vi "DetermineSpeedCap.vi"(2 "Speed Cap Decceleration Limit (/s)":dbl=0.25, 3 "Driver Profile Doesn't Want to Shift":bool, 4 "Master State":T1(ring)) -> (0 "Speed Cap [0,1]":dbl)   [LabVIEW 2020]
doc: "Determines the speed cap for the swerve drive based on the control inputs and master alarms. This includes forcing the robot into low gear."
uses:
  GlobalDriverStationCommands.vi
  GlobalDrivebase.vi
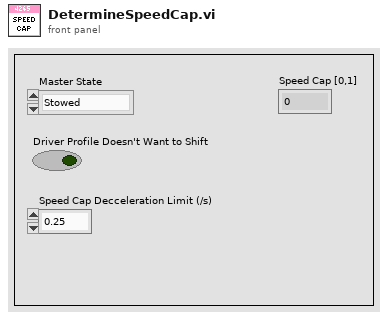
[diagram p1: front panel]
types:
  T1 = enum16{"Stowed", "Balancing", "Scoring", "Hoppering", "Ground", "Shelf"}
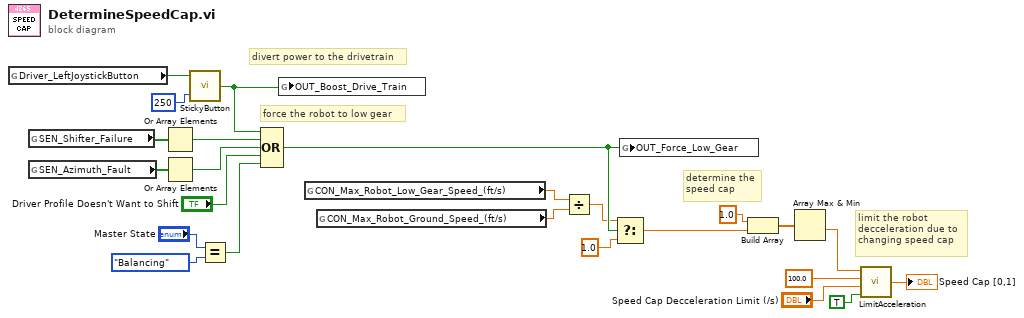
[diagram p0: block diagram]
diagram:
  # "limit the robot\ndecceleration due to\nchanging speed cap"
  # "force the robot to low gear"
  # "determine the\nspeed cap"
  # "divert power to the drivetrain"
  n1 = global read "GlobalDriverStationCommands.vi" "Driver_LeftJoystickButton"() -> (w2:bool)
  n2 = global read "GlobalDrivebase.vi" "SEN_Shifter_Failure"() -> (w22:bool[])
  n3 = global read "GlobalDrivebase.vi" "SEN_Azimuth_Fault"() -> (w21:bool[])
  n4 = Or Array Elements(Boolean array=w22) -> (logical OR=w6:bool)
  n5 = Or Array Elements(Boolean array=w21) -> (logical OR=w5:bool)
  n6 = call "StickyButton.vi"("Time threshold (ms)"=u32 250 ("y"), "Button Input"=w2) -> ("Sticky Button"=w19:bool)
  n7 = Equal?(x="Master State", y=T1."Balancing") -> (x = y?=w1:bool)
  n8 = Compound Arithmetic op=OR(w19, w6, w5, "Driver Profile Doesn't Want to Shift", w1) -> (w20:bool)
  n9 = global write "GlobalDrivebase.vi" "OUT_Boost_Drive_Train"(w19) -> ()
  n10 = global read "GlobalDrivebase.vi" "CON_Max_Robot_Low_Gear_Speed_(ft/s)"() -> (w17:dbl)
  n11 = global read "GlobalDrivebase.vi" "CON_Max_Robot_Ground_Speed_(ft/s)"() -> (w18:dbl)
  n12 = Divide(x=w17, y=w18) -> (x/y=w14:dbl)
  n13 = Select(t=w14, s=w20, f=1.0) -> (s? t:f=w15:dbl)
  n14 = global write "GlobalDrivebase.vi" "OUT_Force_Low_Gear"(w20) -> ()
  n15 = Build Array(1.0 ("element"), w15) -> (w7:dbl[])
  n16 = Array Max & Min(array=w7) -> (min value=w11:dbl)  [unwired: 3 out]
  n17 = call "LimitAcceleration.vi"("Apply Limit"=TRUE, "Decceleration Limit (/s)"="Speed Cap Decceleration Limit (/s)", "Acceleration Limit (/s)"=100.0, "Raw Input"=w11) -> ("Output"=→"Speed Cap [0,1]":dbl)
